vi "Reset Acq Hold Off Counter.vi"(9 "Value":u16, 10 "Reset":bool) -> (1 "Value":u16)   [LabVIEW 2012]
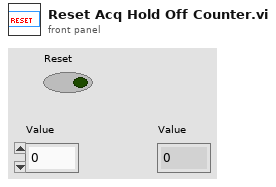
[diagram p1: front panel]
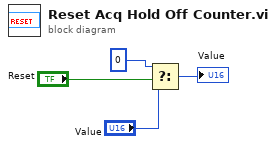
[diagram p0: block diagram]
diagram:
  n1 = Select(t=u16 0, s="Reset", f="Value") -> (s? t:f=→"Value":u16)
